vi "Parse XML Line.vi"(7 "Read past Empty line? (T)":bool=TRUE, 8 "error in (no error)":errorcluster, 11 "XML Refnum in":refnum<file>) -> (0 "error out":errorcluster, 1 "Line Type":T1, 3 "XML Refnum out":refnum<file>)   [LabVIEW 2013, in "XML Parser.lvclass"]
uses:
  XML Parser.lvclass
  XML element Types.ctl
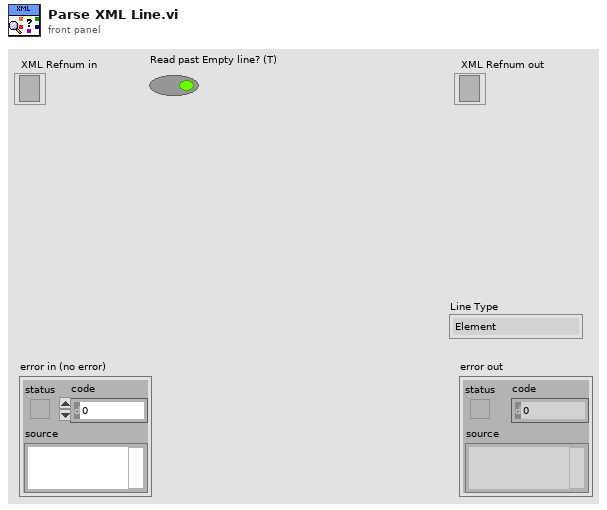
[diagram p1: front panel]
types:
  T1 = typedef "XML Parser.lvclass/XML element Types.ctl" = enum16{"Element", "Comment", "Empty Line"}
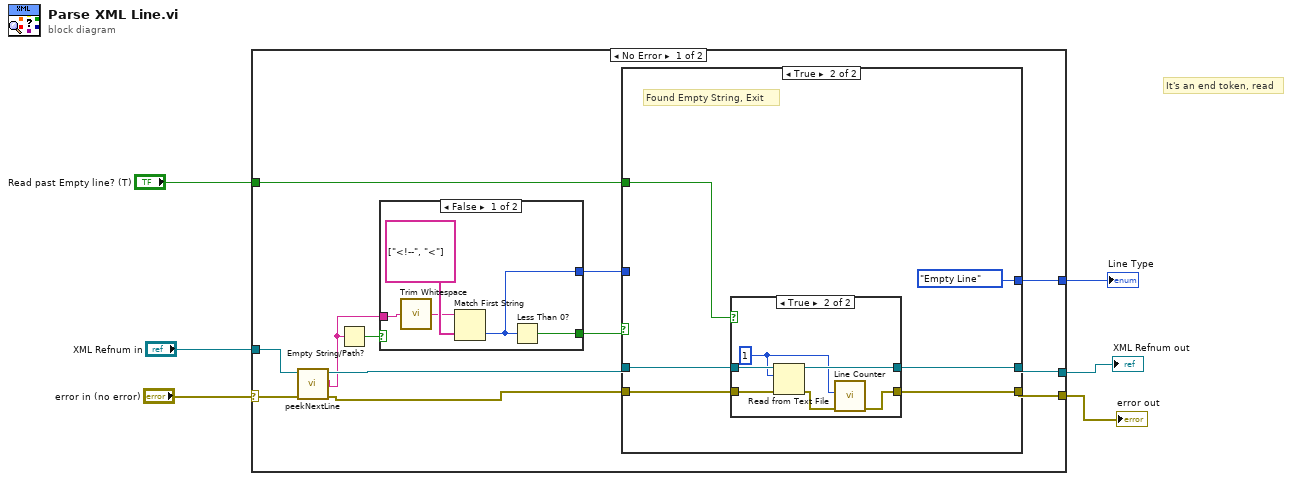
[diagram p0: block diagram]
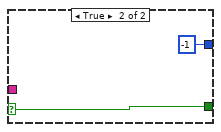
[diagram p2: hidden frame]
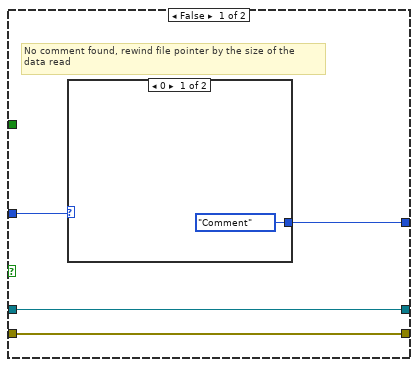
[diagram p3: hidden frame]
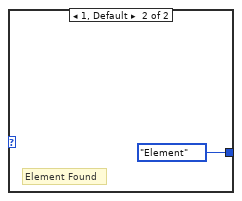
[diagram p4: hidden frame]
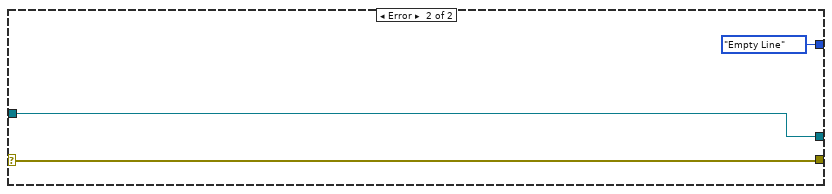
[diagram p6: hidden frame]
diagram:
  # "It's an end token, read"
  n1 = case shown="No Error" "error in (no error)" {
    selector: "error in (no error)" -> [w16 w47]
    tunnel: "XML Refnum in" -> [w15 w48]
    tunnel: [w18 w48] -> w4
    tunnel: [w17 w47] -> w3
    tunnel: "Read past Empty line? (T)" -> [w10 _]
    tunnel: [w9 XML_element_Types."Empty Line" ("Line Type")] -> w1
    frame No Error {
      n2 = call "peekNextLine.vi"("error in"=w16, "file* in"=w15) -> ("error out"=w7:errorcluster, "nextLine"=w11:string, "file* out"=w14:refnum<file>)  [unwired: 7 in]
      n3 = Empty String/Path?(string/path=w11) -> (empty?=w12:bool)
      n4 = case shown="False" w12 {
        selector: w12 -> [_ w25]
        tunnel: [w22 w25] -> w13
        tunnel: w11 -> [w21 _]
        tunnel: [w19 -1 ("index")] -> w8
        frame False {
          n5 = call <vilib>:"Trim Whitespace.vi"("string"=w21) -> ("trimmed string"=w20:string)  [unwired: 1 in]
          n6 = Match First String(2:string[] ["<!--", "<"] ("delimiters (\\s,\\t,\\r,\\n)"), 3:w20) -> (0:w19:i32)  [unwired: 1 out]
          n7 = Less Than 0?(x=w19) -> (x < 0?=w22:bool)
        }
        frame True {
        }
      }
      n8 = case shown="True" w13 {
        tunnel: w14 -> [w29 w37]
        tunnel: w7 -> [w28 w36]
        tunnel: [w29 w35] -> w18
        tunnel: [w28 w34] -> w17
        tunnel: w10 -> [_ w33]
        tunnel: [w26 XML_element_Types."Empty Line" ("Line Type")] -> w9
        tunnel: w8 -> [w27 _]
        frame False {
          # "No comment found, rewind file pointer by the size of the\ndata read"
          n9 = case shown="0" w27 {
            tunnel: [XML_element_Types."Comment" ("Line Type") XML_element_Types."Element" ("Line Type")] -> w26
            frame 0 {
            }
            frame 1, Default {
              # "Element Found"
            }
          }
        }
        frame True {
          # "Found Empty String, Exit"
          n10 = case shown="True" w33 {
            tunnel: w37 -> [w39 w45]
            tunnel: w36 -> [w38 w44]
            tunnel: [w39 w43] -> w35
            tunnel: [w38 w40] -> w34
            frame False {
            }
            frame True {
              w41 = 1 ("count")
              n11 = Read from Text File(file (use dialog)=w45, count=w41, error in=w44) -> (refnum out=w43:refnum<file>, error out=w42:errorcluster)  [unwired: 1 in, 2 out]
              n12 = call "Line Counter.vi"("error in (no error)"=w42, "# of lines to increment (1)"=w41) -> ("error out"=w40:errorcluster)  [unwired: 8 in, 1 out]
            }
          }
        }
      }
    }
    frame Error {
    }
  }
  "XML Refnum out" <- w4
  "error out" <- w3
  "Line Type" <- w1
